vi "getStateName.vi"(9 "error in (no error)":errorcluster, 11 "state in":refnum<class "state.lvclass">) -> (1 "error out":errorcluster, 2 "State Name":string, 3 "state out":refnum<class "state.lvclass">)   [LabVIEW 2020, in "eos.lvlib" / "state.lvclass"]
uses:
  state.lvclass
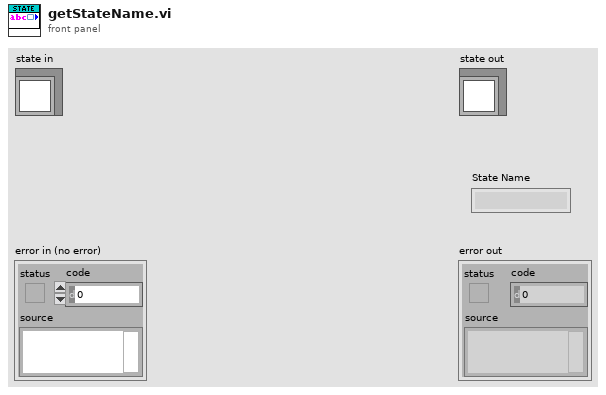
[diagram p1: front panel]
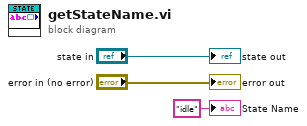
[diagram p0: block diagram]
diagram:
  "error out" <- "error in (no error)"
  "state out" <- "state in"
  "State Name" <- "idle" ("State Name")
